vi "Read First Call.vi"(8 "error in (no error)":errorcluster, 11 "STEP in":refnum<class "STEP.lvclass">) -> (0 "error out":errorcluster, 2 "First Call?":bool, 3 "STEP out":refnum<class "STEP.lvclass">)   [LabVIEW 2018, in "Sequence Composition.lvlib" / "STEP.lvclass"]
uses:
  STEP.lvclass
  STEP.lvclass/STEP.ctl
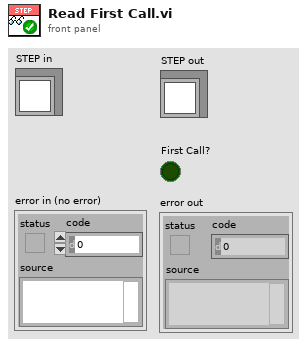
[diagram p1: front panel]
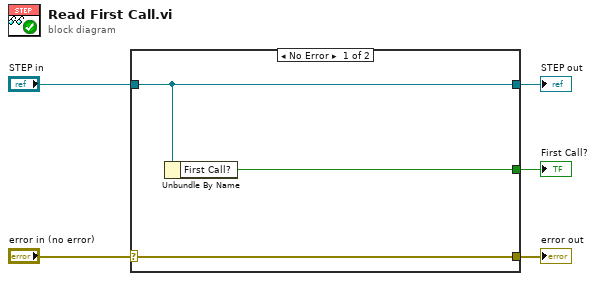
[diagram p0: block diagram]
diagram:
  n1 = case shown="No Error" "error in (no error)" {
    selector: "error in (no error)" -> [w8 w9]
    tunnel: [w8 w9] -> w4
    tunnel: [w7 w10] -> w2
    tunnel: "STEP in" -> [w7 w10]
    tunnel: [w6 _] -> w1
    frame No Error {
      n2 = Unbundle By Name(w7) -> ("First Call?"=w6:bool)
    }
    frame Error {
    }
  }
  "error out" <- w4
  "STEP out" <- w2
  "First Call?" <- w1
